vi "ChirpConvDsbAM.vi"(6 "Modulation Index":dbl(slide) scale=0.0..1.0) -> ()   [LabVIEW 2011]
uses:
  <vilib>/measure/NI_MABase.lvlib
  <vilib>/Analysis/NI_AALBase.lvlib
panel:
  out "Waveform Graph Demodulated":dynamicdata(graph)
  out "Waveform Graph Modulated":waveform(dbl)(graph)
  out "Waveform Graph":waveform(dbl)(graph)
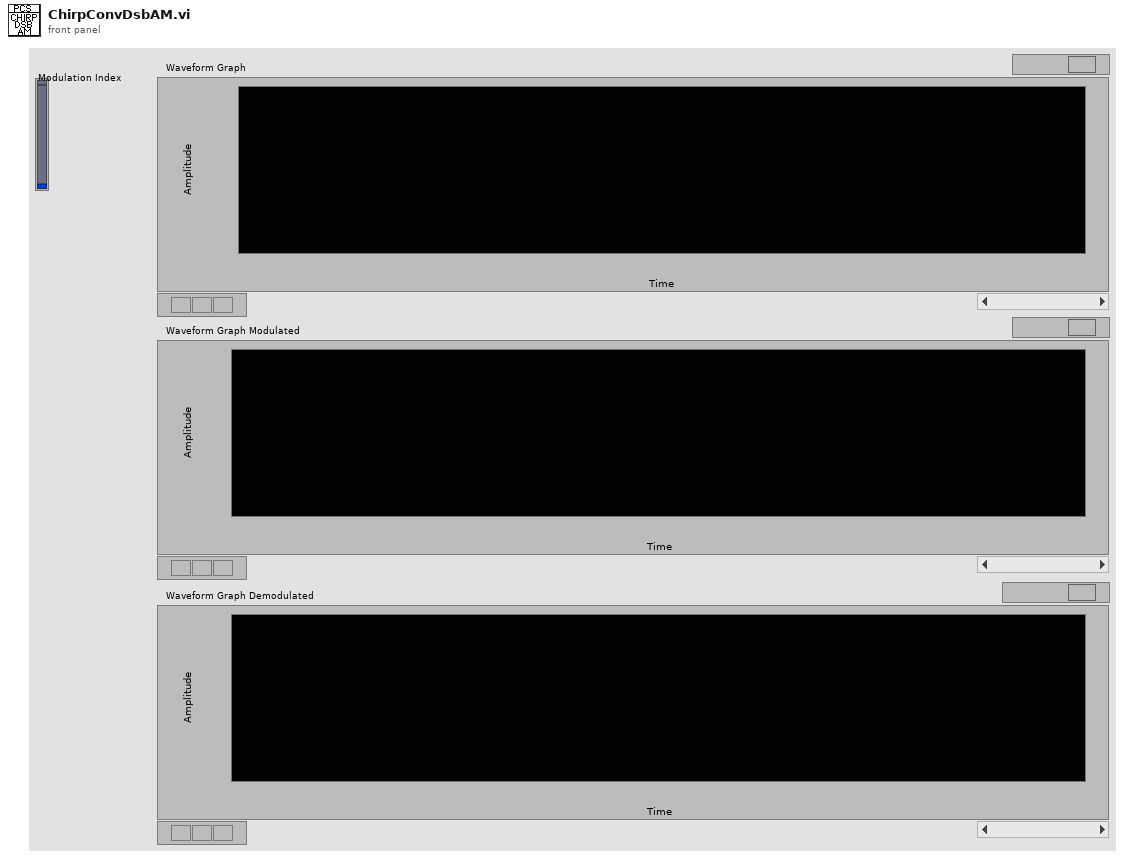
[diagram p1: front panel]
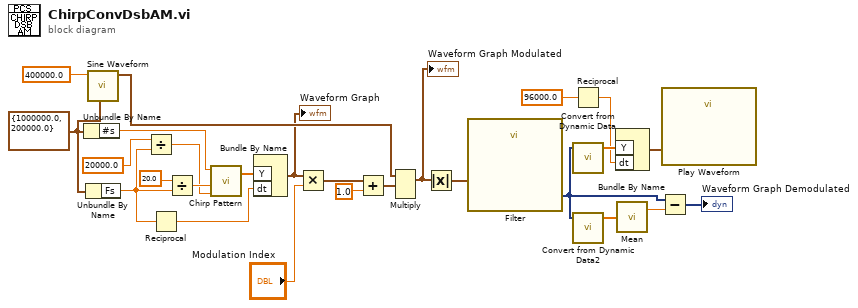
[diagram p0: block diagram]
diagram:
  w6 = cluster{"Fs":dbl, "#s":dbl} {"Fs"=1000000.0, "#s"=200000.0} ("sampling info")
  n1 = Unbundle By Name(w6) -> ("#s"=w15:dbl)
  n2 = Unbundle By Name(w6) -> ("Fs"=w16:dbl)
  n3 = call <vilib>:"Sine Waveform.vi"("sampling info"=w6, "frequency"=400000.0 ("Carrier Freq")) -> ("signal out"=w23:waveform(dbl))  [unwired: 8 in, 1 out]
  n4 = Divide(x=20000.0 ("f2"), y=w16) -> (x/y=w17:dbl)
  n5 = Reciprocal(x=w16) -> (1/x=w5:dbl)
  n6 = Divide(x=20.0 ("f1"), y=w16) -> (x/y=w18:dbl)
  n7 = call <vilib>:"Chirp Pattern.vi"("f2"=w17, "f1"=w18, "samples"=w15) -> ("Chirp Pattern"=w10:dbl[])  [unwired: 1 in, 1 out]
  n8 = Bundle By Name("Y"=w10, "dt"=w5) -> (w9:waveform(dbl))  [unwired: 1 in]
  "Waveform Graph" <- w9
  n9 = Multiply(x=w9, y="Modulation Index") -> (x*y=w26:waveform(dbl))
  n10 = Add(x=w26, y=1.0) -> (x+y=w24:waveform(dbl))
  n11 = Multiply(1:w24, 2:w23) -> (0:w3:waveform(dbl))  [unwired: 1 in, 1 out]
  "Waveform Graph Modulated" <- w3
  n12 = Absolute Value(x=w3) -> (abs(x)=w14:waveform(dbl))
  n13 = call "Filter"("Signal"=w14) -> ("Filtered Signal"=w2:dynamicdata)  [unwired: 9 in, 1 out]
  n14 = Reciprocal(x=96000.0) -> (1/x=w4:dbl)
  n15 = call "Convert from Dynamic Data"("Dynamic Data Type"=w2) -> ("Array"=w7:dbl[])  [unwired: 3 in]
  n16 = call "Convert from Dynamic Data2"("Dynamic Data Type"=w2) -> ("Array"=w1:dbl[])  [unwired: 3 in]
  n17 = Bundle By Name("Y"=w7, "dt"=w4) -> (w8:waveform(dbl))  [unwired: 1 in]
  n18 = call <vilib>:"Mean.vi"("X"=w1) -> ("mean"=w13:dbl)  [unwired: 1 out]
  n19 = Subtract(x=w2, y=w13) -> (x-y=→"Waveform Graph Demodulated":dynamicdata)
  n20 = call "Play Waveform"("Data"=w8) -> ()  [unwired: 18 in, 1 out]
